vi "subtractBackground.vi"(6 "Color Plane":i32(ring)=1 items=["Red", "Green", "Blue", "Hue", "Saturation", "Luminance", "Value", "Intensity"], 7 "subtraction result":T1, 8 "error IO":errorcluster, 9 "downsampling":i32=24, 10 "saveBG":bool, 11 "processed image":T1) -> (0 "error out":errorcluster, 3 "processed image out":T1)   [LabVIEW 2012]
uses:
  <vilib>/vision/Image Controls.llb/IMAQ Image.ctl
  GlobalBaslerCamera.vi
  <vilib>/vision/NI_Vision_Development_Module.lvlib
  <resource>/objmgr/IMAQImage.rc
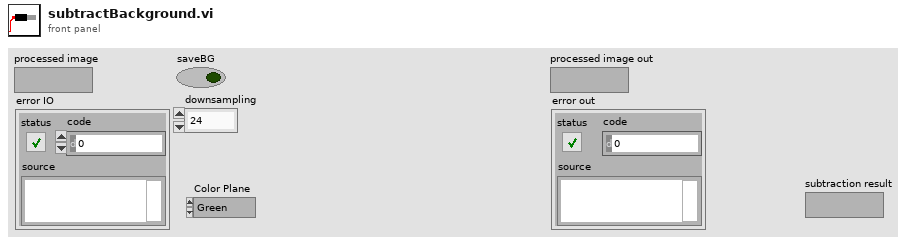
[diagram p1: front panel]
types:
  T1 = typedef "IMAQ Image.ctl" = refnum<image>
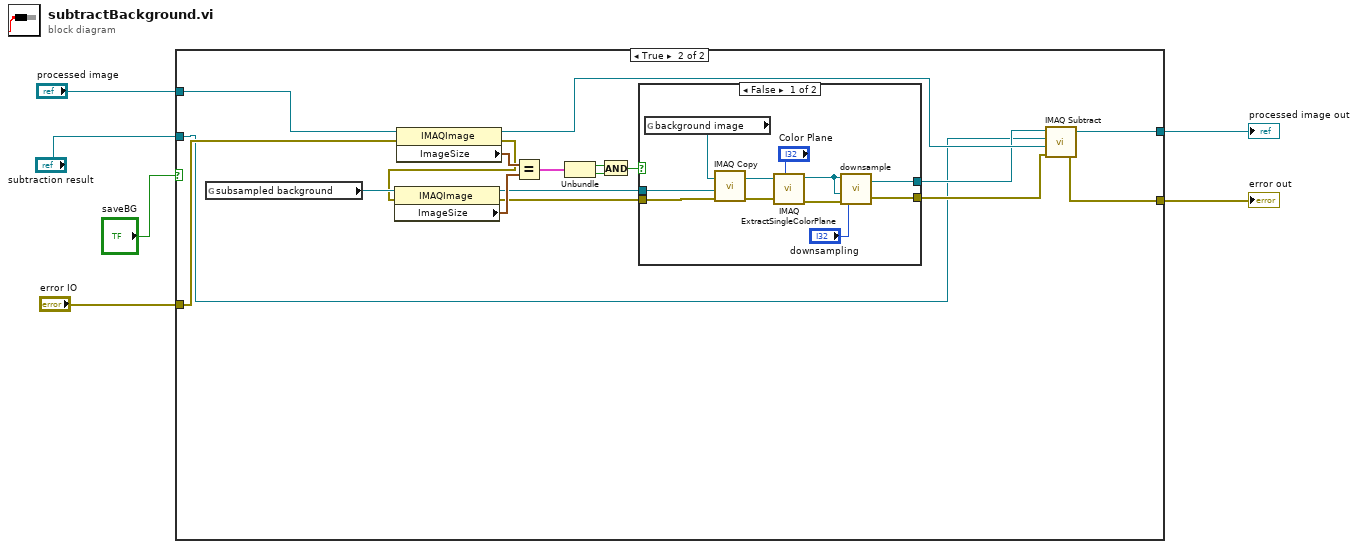
[diagram p0: block diagram]
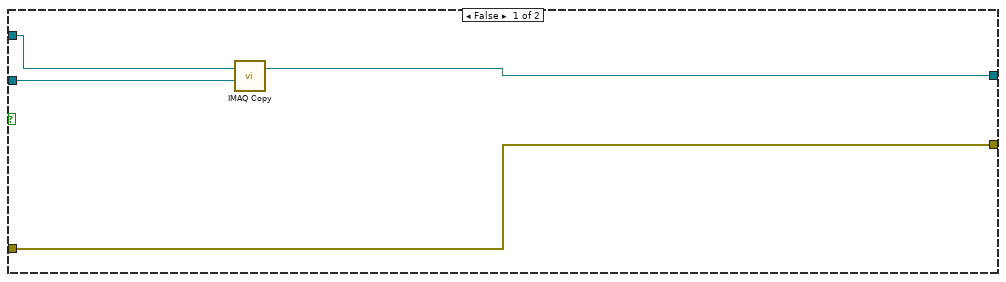
[diagram p2: hidden frame]
diagram:
  n1 = case shown="True" "saveBG" {
    tunnel: "processed image" -> [w8 w25]
    tunnel: [w9 w28] -> w3
    tunnel: "error IO" -> [w10 w13]
    tunnel: [w10 w27] -> w2
    tunnel: "subtraction result" -> [w7 w11]
    frame False {
      n2 = call "IMAQ Copy"("Image Dst"=w7, "Image Src"=w8) -> ("Image Dst Out"=w9:T1)  [unwired: 4 in, 1 out]
    }
    frame True {
      n3 = global read "GlobalBaslerCamera.vi" "subsampled background"() -> (w26:T1)
      n4 = property class="IMAQImage"(reference=w25, error in=w13) -> (reference out=w18:T1, error out=w14:errorcluster, "ImageSize"=w24:cluster{"x":i32, "y":i32})
      n5 = property class="IMAQImage"(reference=w26, error in=w14) -> (reference out=w17:T1, error out=w15:errorcluster, "ImageSize"=w23:cluster{"x":i32, "y":i32})
      n6 = Equal?(x=w24, y=w23) -> (x = y?=w22:cluster{"x":bool, "y":bool})
      n7 = Unbundle(w22) -> ("x"=w21:bool, "y"=w20:bool)
      n8 = And(x=w21, y=w20) -> (x .and. y?=w19:bool)
      n9 = case shown="False" w19 {
        tunnel: w17 -> [w39 w41]
        tunnel: [w38 w41] -> w16
        tunnel: w15 -> [w35 w40]
        tunnel: [w34 w40] -> w12
        frame False {
          n10 = global read "GlobalBaslerCamera.vi" "background image"() -> (w36:T1)
          n11 = call "IMAQ Copy"("error in (no error)"=w35, "Image Dst"=w39, "Image Src"=w36) -> ("error out"=w32:errorcluster, "Image Dst Out"=w33:T1)  [unwired: 3 in]
          n12 = call "IMAQ ExtractSingleColorPlane"("Color Plane"="Color Plane", "error in (no error)"=w32, "Image Src"=w33) -> ("error out"=w31:errorcluster, "Image Dst Out"=w30:T1)  [unwired: 7 in]
          n13 = call "downsample.vi"("error in"=w31, "img dst"=w30, "downsampling"="downsampling", "img src"=w30) -> ("error out"=w34:errorcluster, "Image Dst Out"=w38:T1)
        }
        frame True {
        }
      }
      n14 = call "IMAQ Subtract"("Image Src A"=w16, "Image Dst"=w11, "Image Src B"=w18, "error in (no error)"=w12) -> ("Image Dst Out"=w28:T1, "error out"=w27:errorcluster)  [unwired: 3 in]
    }
  }
  "processed image out" <- w3
  "error out" <- w2
